vi "get_value.vi"(8 "error in (no error)":errorcluster, 10 "channel":dbl, 11 "LakeShore336 in":refnum<class "Lakeshore_336.lvclass">) -> (0 "error out":errorcluster, 2 "value":string, 3 "LakeShore336 out":refnum<class "Lakeshore_336.lvclass">)   [LabVIEW 2018, in "Lakeshore_336.lvclass"]
doc: "the vi reads the value (pressure, temp etc etc) from the instrument"
uses:
  Lakeshore_336.lvclass
  instrument.lvclass
  Drivers/Lake Shore 336/Lake Shore 336.lvlib
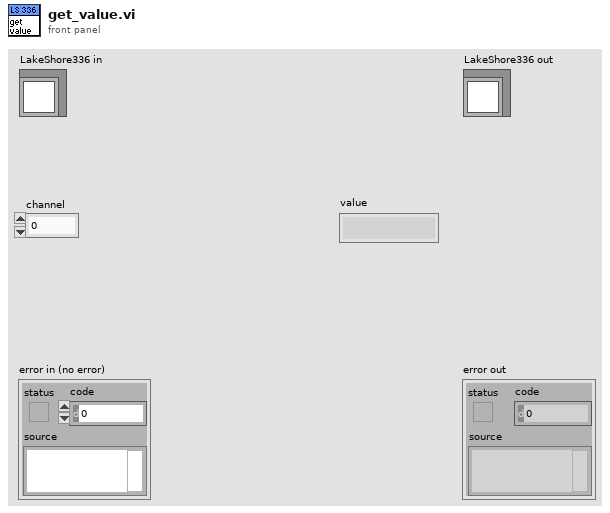
[diagram p1: front panel]
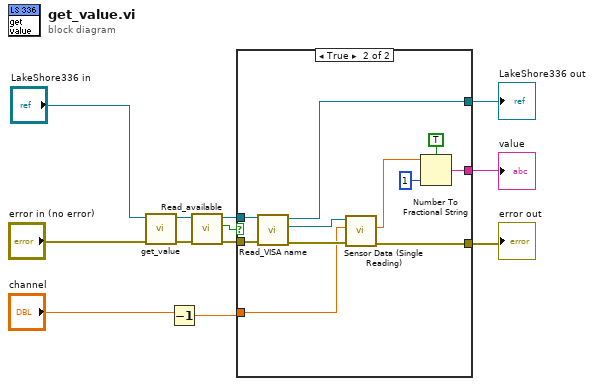
[diagram p0: block diagram]
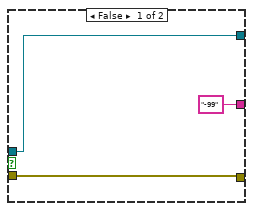
[diagram p2: hidden frame]
diagram:
  n1 = call-parent "get_value.vi"("error in (no error)"="error in (no error)", "instrument in"="LakeShore336 in") -> ("error out"=w6:errorcluster, "instrument out"=w7:refnum<class "Lakeshore_336.lvclass">)  [unwired: 7 in, 1 out]
  n2 = Decrement(x="channel") -> (x-1=w1:dbl)
  n3 = call-dynamic "Read_available.vi"("error in (no error)"=w6, "instrument in"=w7) -> ("error out"=w4:errorcluster, "available?"=w3:bool, "instrument out"=w5:refnum<class "Lakeshore_336.lvclass">)  [unwired: 7 in]
  n4 = case shown="True" w3 {
    tunnel: [w15 w26] -> w10
    tunnel: w1 -> [_ w23]
    tunnel: [w14 w22] -> w9
    tunnel: ["-99" w21] -> w8
    tunnel: w5 -> [w15 w18]
    tunnel: w4 -> [w14 w17]
    frame False {
    }
    frame True {
      n5 = call-dynamic "Read_VISA name.vi"("error in (no error)"=w17, "instrument in"=w18) -> ("error out"=w24:errorcluster, "VISA resource name"=w25:refnum<visa-resource-name>, "instrument out"=w26:refnum<class "Lakeshore_336.lvclass">)  [unwired: 7 in]
      n6 = call "Sensor Data (Single Reading).vi"("error in (no error)"=w24, "Input (0:A)"=w23, "VISA resource name"=w25) -> ("error out"=w22:errorcluster, "Sensor Data"=w20:dbl)  [unwired: 6 in, 1 out]
      n7 = Number To Fractional String(use system decimal point (T)=TRUE, number=w20, precision (6)=i16 1) -> (F-format string=w21:string)  [unwired: 1 in]
    }
  }
  "error out" <- w9
  "LakeShore336 out" <- w10
  "value" <- w8
